vi "IS Generate Random Bucket Key.vi"() -> (3 "string":string)   [LabVIEW 2013]
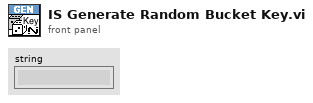
[diagram p1: front panel]
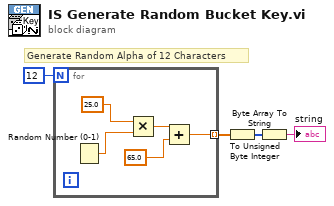
[diagram p0: block diagram]
diagram:
  # "Generate Random Alpha of 12 Characters"
  n1 = for {
    N: 12 -> [_]
    tunnel: [w5] -> w2 mode=indexing
    n2 = Random Number (0-1)() -> (number: 0 to 1=w8:dbl)
    n3 = Multiply(x=25.0, y=w8) -> (x*y=w7:dbl)
    n4 = Add(x=w7, y=65.0) -> (x+y=w5:dbl)
  }
  n5 = To Unsigned Byte Integer(number=w2) -> (unsigned 8bit integer=w3:u8[])
  n6 = Byte Array To String(unsigned byte array=w3) -> (string=→"string":string)
